vi "Mouse click event.vi"(8 "error in":errorcluster, 10 "Mouse Click":T1(ring)) -> (0 "error out":errorcluster)   [LabVIEW 2012]
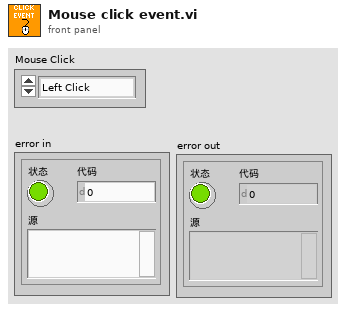
[diagram p1: front panel]
types:
  T1 = enum16{"Left Click", "Left dbClick", "Right Click", "Right dbClick", "Middle Click", "Middle dbClick"}
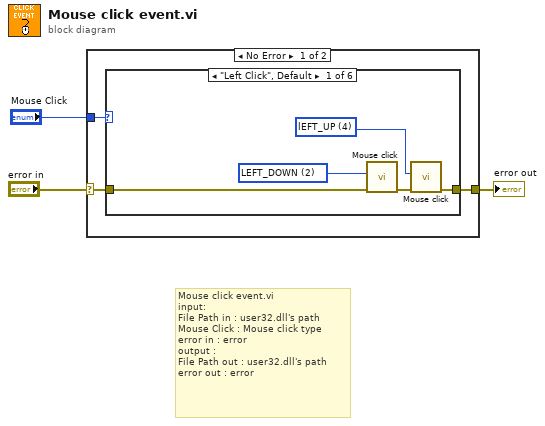
[diagram p0: block diagram]
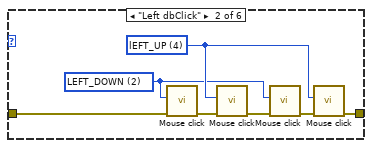
[diagram p2: hidden frame]
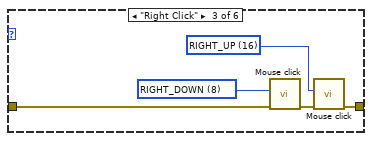
[diagram p3: hidden frame]
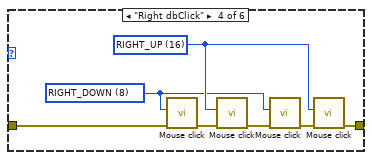
[diagram p4: hidden frame]
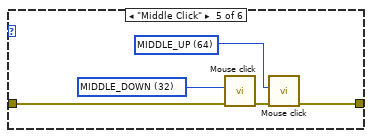
[diagram p5: hidden frame]
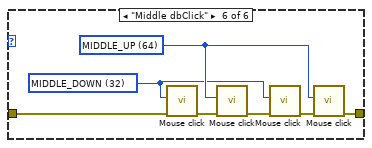
[diagram p6: hidden frame]
diagram:
  # "Mouse click event.vi\ninput:\nFile Path in : user32.dll's path\nMouse Click : Mouse click type\nerror in : error\noutput : \nFile Path out : user32.dll's path\nerror out : error"
  n1 = case shown="No Error" "error in" {
    selector: "error in" -> [w5 w43]
    tunnel: [w6 w43] -> w3
    tunnel: "Mouse Click" -> [w4 _]
    frame No Error {
      n2 = case shown="\"Left Click\", Default" w4 {
        tunnel: w5 -> [w11 w18 w23 w29 w35 w42]
        tunnel: [w9 w14 w21 w26 w33 w38] -> w6
        frame "Left Click", Default {
          w7 = u32 2 items=["MOVE"=1, "LEFT_DOWN"=2, "lEFT_UP"=4, "RIGHT_DOWN"=8, "RIGHT_UP"=16, "MIDDLE_DOWN"=32, "MIDDLE_UP"=64, "MOUSE_WHEEL"=128, "ABSOLUTE"=32768] ("Mouse_Event dwFlags")
          w8 = u32 4 items=["MOVE"=1, "LEFT_DOWN"=2, "lEFT_UP"=4, "RIGHT_DOWN"=8, "RIGHT_UP"=16, "MIDDLE_DOWN"=32, "MIDDLE_UP"=64, "MOUSE_WHEEL"=128, "ABSOLUTE"=32768] ("Mouse_Event dwFlags")
          n3 = call "Mouse click.vi"("error in"=w11, "Mouse click"=w7) -> ("error out"=w10:errorcluster)  [unwired: 9 in]
          n4 = call "Mouse click.vi"("error in"=w10, "Mouse click"=w8) -> ("error out"=w9:errorcluster)  [unwired: 9 in]
        }
        frame "Left dbClick" {
          w12 = u32 2 items=["MOVE"=1, "LEFT_DOWN"=2, "lEFT_UP"=4, "RIGHT_DOWN"=8, "RIGHT_UP"=16, "MIDDLE_DOWN"=32, "MIDDLE_UP"=64, "MOUSE_WHEEL"=128, "ABSOLUTE"=32768] ("Mouse_Event dwFlags")
          w13 = u32 4 items=["MOVE"=1, "LEFT_DOWN"=2, "lEFT_UP"=4, "RIGHT_DOWN"=8, "RIGHT_UP"=16, "MIDDLE_DOWN"=32, "MIDDLE_UP"=64, "MOUSE_WHEEL"=128, "ABSOLUTE"=32768] ("Mouse_Event dwFlags")
          n5 = call "Mouse click.vi"("error in"=w18, "Mouse click"=w12) -> ("error out"=w17:errorcluster)  [unwired: 9 in]
          n6 = call "Mouse click.vi"("error in"=w17, "Mouse click"=w13) -> ("error out"=w16:errorcluster)  [unwired: 9 in]
          n7 = call "Mouse click.vi"("error in"=w16, "Mouse click"=w12) -> ("error out"=w15:errorcluster)  [unwired: 9 in]
          n8 = call "Mouse click.vi"("error in"=w15, "Mouse click"=w13) -> ("error out"=w14:errorcluster)  [unwired: 9 in]
        }
        frame "Right Click" {
          w19 = u32 8 items=["MOVE"=1, "LEFT_DOWN"=2, "lEFT_UP"=4, "RIGHT_DOWN"=8, "RIGHT_UP"=16, "MIDDLE_DOWN"=32, "MIDDLE_UP"=64, "MOUSE_WHEEL"=128, "ABSOLUTE"=32768] ("Mouse_Event dwFlags")
          w20 = u32 16 items=["MOVE"=1, "LEFT_DOWN"=2, "lEFT_UP"=4, "RIGHT_DOWN"=8, "RIGHT_UP"=16, "MIDDLE_DOWN"=32, "MIDDLE_UP"=64, "MOUSE_WHEEL"=128, "ABSOLUTE"=32768] ("Mouse_Event dwFlags")
          n9 = call "Mouse click.vi"("error in"=w23, "Mouse click"=w19) -> ("error out"=w22:errorcluster)  [unwired: 9 in]
          n10 = call "Mouse click.vi"("error in"=w22, "Mouse click"=w20) -> ("error out"=w21:errorcluster)  [unwired: 9 in]
        }
        frame "Right dbClick" {
          w24 = u32 8 items=["MOVE"=1, "LEFT_DOWN"=2, "lEFT_UP"=4, "RIGHT_DOWN"=8, "RIGHT_UP"=16, "MIDDLE_DOWN"=32, "MIDDLE_UP"=64, "MOUSE_WHEEL"=128, "ABSOLUTE"=32768] ("Mouse_Event dwFlags")
          w25 = u32 16 items=["MOVE"=1, "LEFT_DOWN"=2, "lEFT_UP"=4, "RIGHT_DOWN"=8, "RIGHT_UP"=16, "MIDDLE_DOWN"=32, "MIDDLE_UP"=64, "MOUSE_WHEEL"=128, "ABSOLUTE"=32768] ("Mouse_Event dwFlags")
          n11 = call "Mouse click.vi"("error in"=w29, "Mouse click"=w24) -> ("error out"=w28:errorcluster)  [unwired: 9 in]
          n12 = call "Mouse click.vi"("error in"=w28, "Mouse click"=w25) -> ("error out"=w30:errorcluster)  [unwired: 9 in]
          n13 = call "Mouse click.vi"("error in"=w30, "Mouse click"=w24) -> ("error out"=w27:errorcluster)  [unwired: 9 in]
          n14 = call "Mouse click.vi"("error in"=w27, "Mouse click"=w25) -> ("error out"=w26:errorcluster)  [unwired: 9 in]
        }
        frame "Middle Click" {
          w31 = u32 32 items=["MOVE"=1, "LEFT_DOWN"=2, "lEFT_UP"=4, "RIGHT_DOWN"=8, "RIGHT_UP"=16, "MIDDLE_DOWN"=32, "MIDDLE_UP"=64, "MOUSE_WHEEL"=128, "ABSOLUTE"=32768] ("Mouse_Event dwFlags")
          w32 = u32 64 items=["MOVE"=1, "LEFT_DOWN"=2, "lEFT_UP"=4, "RIGHT_DOWN"=8, "RIGHT_UP"=16, "MIDDLE_DOWN"=32, "MIDDLE_UP"=64, "MOUSE_WHEEL"=128, "ABSOLUTE"=32768] ("Mouse_Event dwFlags")
          n15 = call "Mouse click.vi"("error in"=w35, "Mouse click"=w31) -> ("error out"=w34:errorcluster)  [unwired: 9 in]
          n16 = call "Mouse click.vi"("error in"=w34, "Mouse click"=w32) -> ("error out"=w33:errorcluster)  [unwired: 9 in]
        }
        frame "Middle dbClick" {
          w36 = u32 32 items=["MOVE"=1, "LEFT_DOWN"=2, "lEFT_UP"=4, "RIGHT_DOWN"=8, "RIGHT_UP"=16, "MIDDLE_DOWN"=32, "MIDDLE_UP"=64, "MOUSE_WHEEL"=128, "ABSOLUTE"=32768] ("Mouse_Event dwFlags")
          w37 = u32 64 items=["MOVE"=1, "LEFT_DOWN"=2, "lEFT_UP"=4, "RIGHT_DOWN"=8, "RIGHT_UP"=16, "MIDDLE_DOWN"=32, "MIDDLE_UP"=64, "MOUSE_WHEEL"=128, "ABSOLUTE"=32768] ("Mouse_Event dwFlags")
          n17 = call "Mouse click.vi"("error in"=w42, "Mouse click"=w36) -> ("error out"=w41:errorcluster)  [unwired: 9 in]
          n18 = call "Mouse click.vi"("error in"=w41, "Mouse click"=w37) -> ("error out"=w40:errorcluster)  [unwired: 9 in]
          n19 = call "Mouse click.vi"("error in"=w40, "Mouse click"=w36) -> ("error out"=w39:errorcluster)  [unwired: 9 in]
          n20 = call "Mouse click.vi"("error in"=w39, "Mouse click"=w37) -> ("error out"=w38:errorcluster)  [unwired: 9 in]
        }
      }
    }
    frame Error {
    }
  }
  "error out" <- w3
